vi "Read Transport Type .vi"(8 "error in (no error)":errorcluster, 11 "WAMP Client in":refnum<class "WAMP Client.lvclass">) -> (0 "error out":errorcluster, 2 "Transport Type":T1, 3 "WAMP Client out":refnum<class "WAMP Client.lvclass">)   [LabVIEW 2021, in "wamplv.lvlib" / "WAMP Client.lvclass"]
uses:
  WAMP Client.lvclass
  WAMP Client.lvclass/WAMP Client.ctl
  API/TypeDefs/Transport Type.ctl
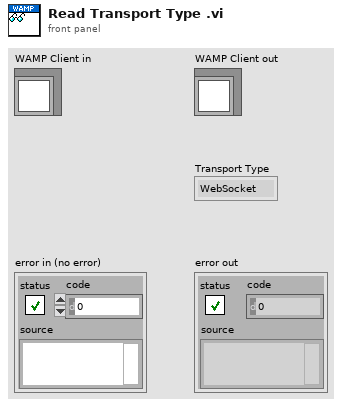
[diagram p1: front panel]
types:
  T1 = typedef "wamplv.lvlib/WAMP Client.lvclass/Transport Type.ctl" = enum16{"WebSocket", "RawSocket TCP"}
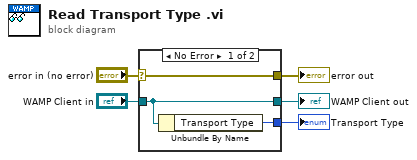
[diagram p0: block diagram]
diagram:
  n1 = case shown="No Error" "error in (no error)" {
    selector: "error in (no error)" -> [w8 w9]
    tunnel: [w8 w9] -> w4
    tunnel: [w7 w10] -> w2
    tunnel: "WAMP Client in" -> [w7 w10]
    tunnel: [w6 _] -> w1
    frame No Error {
      n2 = Unbundle By Name(w7) -> ("Transport Type"=w6:T1)
    }
    frame Error {
    }
  }
  "error out" <- w4
  "WAMP Client out" <- w2
  "Transport Type" <- w1
